vi "p2.2.vi"() -> ()   [LabVIEW 2020]
uses:
  <vilib>/Analysis/NI_AALBase.lvlib
panel:
  out "Periodo de muestreo":dbl
  in  "Frecuencia de muestreo":dbl
  in  "Frecuencia del tono":dbl
  in  "samples":i32=128
  in  "amplitude":dbl=1.0 format="%0.2f"
  out "Waveform Graph":dbl[](graph)
  out "frecuencia labview (ciclos/muestra)":dbl
  out "frecuencia radianes":dbl
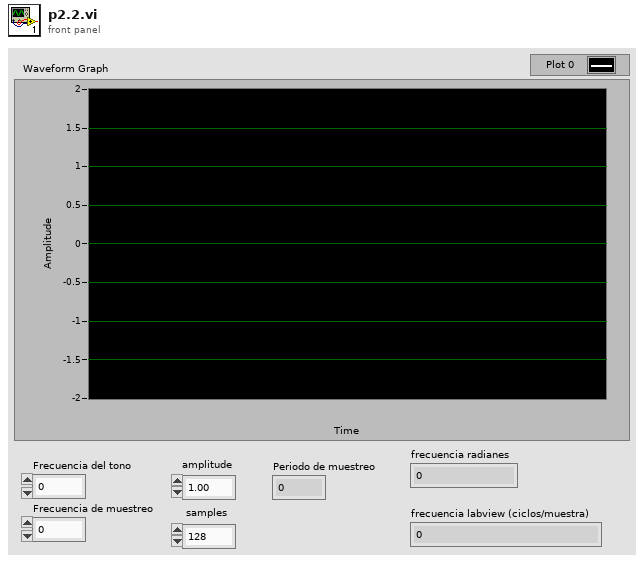
[diagram p1: front panel]
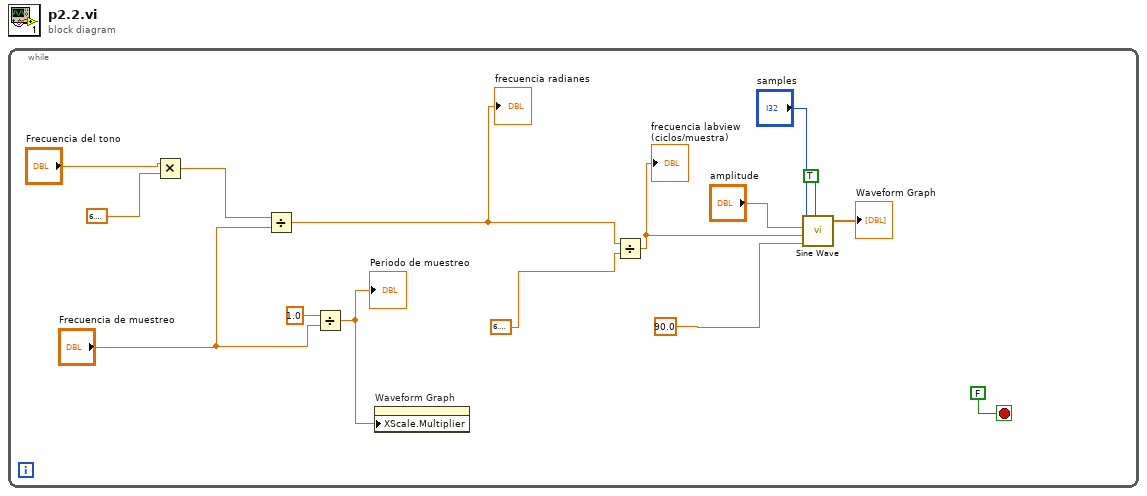
[diagram p0: block diagram]
diagram:
  n1 = while {
    stop <- FALSE ("stop") stop-if-true
    n2 = Multiply(x="Frecuencia del tono", y=6.283185307179586) -> (x*y=w6:dbl)
    n3 = Divide(x=w6, y="Frecuencia de muestreo") -> (x/y=w5:dbl)
    "frecuencia radianes" <- w5
    n4 = Divide(x=1.0, y="Frecuencia de muestreo") -> (x/y=w1:dbl)
    "Periodo de muestreo" <- w1
    n5 = property on="Waveform Graph" class="WFGraph (strict)"("XScale.Multiplier"=w1) -> ()  [unwired: 2 in, 2 out]
    n6 = Divide(x=w5, y=6.283185307179586) -> (x/y=w14:dbl)
    "frecuencia labview (ciclos/muestra)" <- w14
    n7 = call <vilib>:"Sine Wave.vi"("samples"="samples", "amplitude"="amplitude", "frequency"=w14, "phase in"=90.0, "reset phase"=TRUE) -> ("sine wave"=→"Waveform Graph":dbl[])  [unwired: 2 out]
  }
